vi "funny average.vi"(10 "in":dbl[](array[numeric])) -> (2 "Out":dbl[](array[numeric]))   [LabVIEW 2020]
panel:
  out "s? t:f":i32
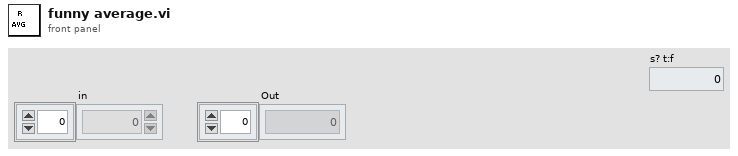
[diagram p1: front panel]
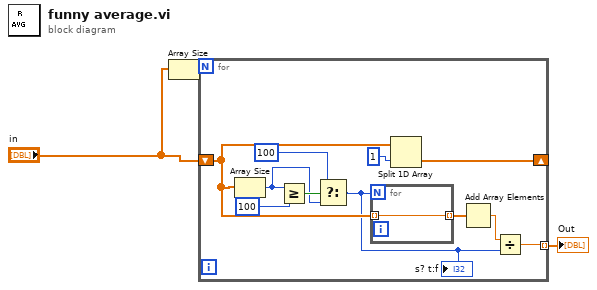
[diagram p0: block diagram]
diagram:
  n1 = Array Size(array="in") -> (size(s)=w3:i32)
  n2 = for {
    N: w3 -> [_]
    shift-right: [w13] -> _
    shift-left: "in" -> [w9]
    tunnel: [w10] -> w1 mode=indexing
    n3 = Array Size(array=w9) -> (size(s)=w5:i32)
    n4 = Greater Or Equal?(x=w5, y=100) -> (x >= y?=w7:bool)
    n5 = Select(t=100, s=w7, f=w5) -> (s? t:f=w4:i32)
    "s? t:f" <- w4
    n6 = for {
      N: w4 -> [_]
      tunnel: w9 -> [w15] mode=indexing
      tunnel: [w15] -> w12 mode=indexing
    }
    n7 = Split 1D Array(array=w9, index=1) -> (second subarray=w13:dbl[])  [unwired: 1 out]
    n8 = Add Array Elements(numeric array=w12) -> (sum=w11:dbl)
    n9 = Divide(x=w11, y=w4) -> (x/y=w10:dbl)
  }
  "Out" <- w1
